vi "var_to_string.vi"(11 "Var Array":string[][](array[string])) -> (3 "VAR string":string)   [LabVIEW 2015, in "oskar_tools.lvlib"]
uses:
  oskar_tools.lvlib
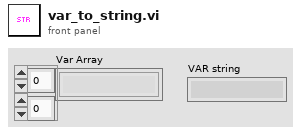
[diagram p1: front panel]
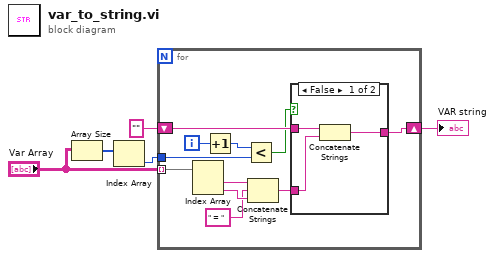
[diagram p0: block diagram]
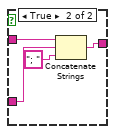
[diagram p2: hidden frame]
diagram:
  n1 = Array Size(array="Var Array") -> (size(s)=w4:i32[])
  n2 = Index Array(array=w4) -> (element=w3:i32)  [unwired: 1 in]
  n3 = for {
    tunnel: "Var Array" -> [w10] mode=indexing
    shift-right: [w16] -> w1
    shift-left: "" ("spreadsheet string") -> [w15]
    tunnel: w3 -> [w7]
    i -> [w9]
    n4 = Index Array(array=w10) -> (element #1=w13:string, element #2=w14:string)  [unwired: 2 in]
    n5 = Increment(x=w9) -> (x+1=w8:i32)
    n6 = Less?(x=w8, y=w7) -> (x < y?=w6:bool)
    n7 = Concatenate Strings(w13, " = " ("string"), w14) -> (w11:string)
    n8 = case shown="False" w6 {
      tunnel: w11 -> [w19 w23]
      tunnel: [w17 w21] -> w16
      tunnel: w15 -> [w18 w20]
      frame False {
        n9 = Concatenate Strings(w18, w19) -> (w17:string)
      }
      frame True {
        n10 = Concatenate Strings(w20, w23, "; " ("string")) -> (w21:string)
      }
    }
  }
  "VAR string" <- w1
